vi "CreateDefectFile.vi"(4 "Region":u16, 7 "Pass rate":dbl format="%.2f", 8 "Defect description list":i32[](array[numeric]), 9 "Bad channel array":i32[](array[numeric]), 10 "No of bad strips":i32, 11 "Filename IN":string) -> (0 "DBfileSaved?":bool, 1 "passed":bool)   [LabVIEW 2018]
uses:
  general_VIs/globals/QC_RunInformation.vi
panel:
  in  "cancel":bool
  in  "create file":bool
  out "% good strips:":dbl format="%.2f"
  out "Passed?":bool
  out "ITk Serial No.:":string
  in  "Bad channel list":i32(listbox)
  # "Write Strip Defect DataBase File"
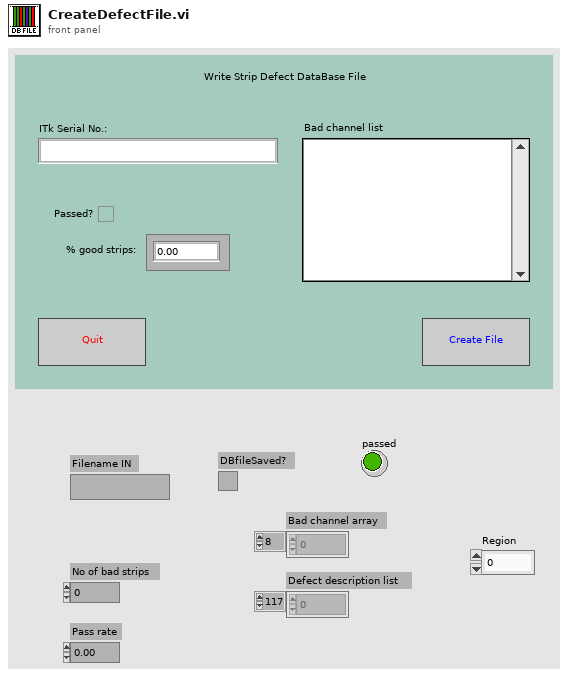
[diagram p1: front panel]
types:
  T1 = cluster{"Institute":string, "Manufacturers":string[], "Devices":string[], "Serialnumbers Lookup DB":string, "Data directory":string, "Backup & screenshot directory":string, "List of known users":string[], "Measurement switch not used":bool, "Measurement Switch":string, "DUT Switch":string, "Rseries IV [MOhm]":string, "Rshunt IV [MOhm]":string, "Rseries CV [MOhm]":string, "DC blocking Cap [µF]":string, "Rseries LCR [MOhm]":string, "Rseries stability [MOhm]":string, "Rshunt stability [MOhm]":string, "Rseries striptest bias [MOhm]":string, "Rseries strip pinhole [MOhm]":string}
  T2 = cluster{"Sensor Serial No.:":string, "Wafer:":string, "Batch:":string, "Manufacturer:":string, "Device Category:":string, "Database Serial No.:":string, "Date Initiated:":string, "Time Initiated:":string, "Test":string, "Probeplan used:":string, "End of Run Status":dbl, "End of Run comment:":string, "User:":string, "Vbias SMU":string, "LCR":string, "Test SMU":string, "Test DMM":string, "Comments":string, "Measurement results":cluster{"IV":string, "CV":string, "Cis":string, "Ris":string, "Stability":string, "PTP":string, "Striptest":string}}
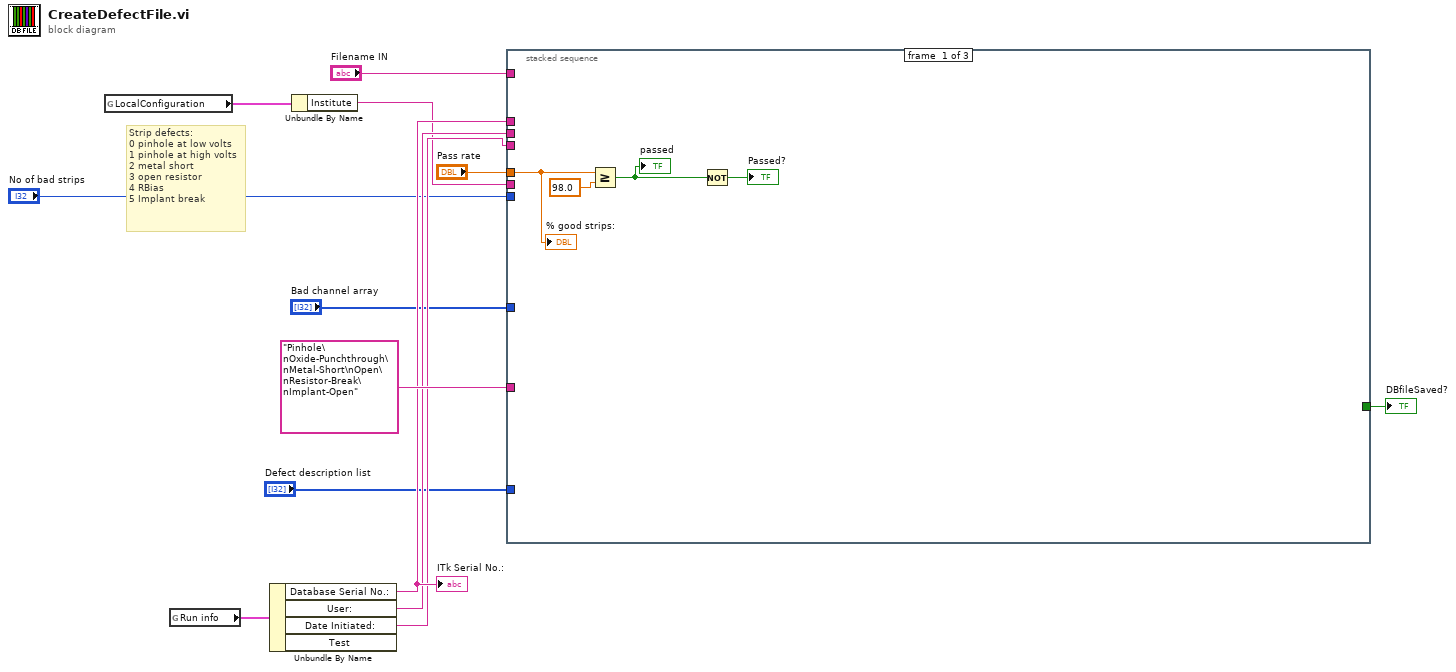
[diagram p0: block diagram]
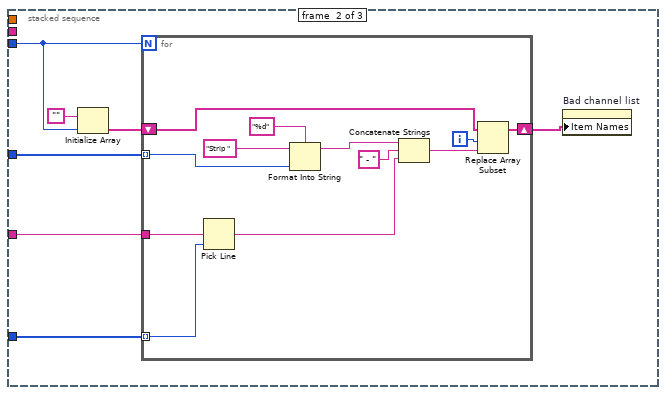
[diagram p2: hidden frame]
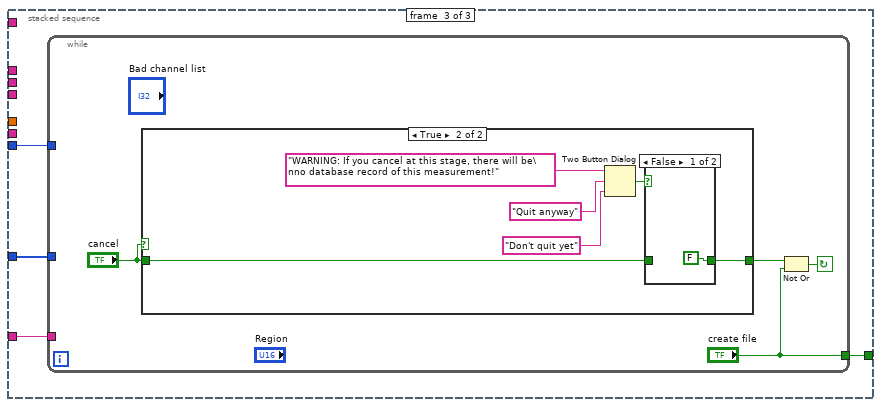
[diagram p3: hidden frame]
diagram:
  # "Strip defects:\n0 pinhole at low volts\n1 pinhole at high volts\n2 metal short\n3 open resistor\n4 RBias\n5 Implant break"
  n1 = global read "QC_RunInformation.vi" "LocalConfiguration"() -> (w2:T1)
  n2 = global read "QC_RunInformation.vi" "Run info"() -> (w12:T2)
  n3 = Unbundle By Name(w12) -> ("Database Serial No.:"=w11:string, "User:"=w10:string, "Date Initiated:"=w9:string)  [unwired: 1 out]
  "ITk Serial No.:" <- w11
  n4 = Unbundle By Name(w2) -> ("Institute"=w1:string)
  n5 = stacked-sequence {
    tunnel: "No of bad strips" -> [_ w18 w39]
    tunnel: "Bad channel array" -> [_ w21 w40]
    tunnel: "Pinhole\nOxide-Punchthrough\nMetal-Short\nOpen\nResistor-Break\nImplant-Open" -> [_ w22 w38]
    tunnel: w11 -> [_ _ _]
    tunnel: w10 -> [_ _ _]
    tunnel: w9 -> [_ _ _]
    tunnel: w1 -> [_ _ _]
    tunnel: [_ _ w37] -> w8
    tunnel: "Filename IN" -> [_ _ _]
    tunnel: "Defect description list" -> [_ w20 _]
    tunnel: "Pass rate" -> [w15 _ _]
    frame #0 {
      n6 = Greater Or Equal?(x=w15, y=98.0) -> (x >= y?=w14:bool)
      "passed" <- w14
      n7 = Not(x=w14) -> (.not. x?=→"Passed?":bool)
      "% good strips:" <- w15
    }
    frame #1 {
      n8 = Initialize Array("", w18) -> (w23:string[])
      n9 = for {
        N: w18 -> [_]
        shift-right: [w31] -> w19
        shift-left: w23 -> [w34]
        tunnel: w21 -> [w25] mode=indexing
        tunnel: w22 -> [w30]
        tunnel: w20 -> [w26] mode=indexing
        i -> [w33]
        n10 = Pick Line(multi-line string=w30, line index=w26) -> (output string=w27:string)  [unwired: 1 in]
        n11 = Format Into String(format string="%d", initial string="Strip ", w25) -> (resulting string=w29:string)  [unwired: 1 in, 1 out]
        n12 = Concatenate Strings(w29, " - ", w27) -> (w32:string)
        n13 = Replace Array Subset(array=w34, new element=w32, index=w33) -> (w31:string[])
      }
      n14 = property on="Bad channel list" class="LstBox (strict)"("Item Names"=w19) -> ()  [unwired: 2 in, 2 out]
    }
    frame #2 {
      n15 = while {
        tunnel: ["create file"] -> w37
        tunnel: w40 -> [_]
        tunnel: w39 -> [_]
        tunnel: w38 -> [_]
        stop <- w44 continue-if-true
        n16 = case shown="True" "cancel" {
          tunnel: [w45 w47] -> w42
          tunnel: "cancel" -> [w45 w46]
          frame False {
          }
          frame True {
            n17 = Two Button Dialog(message="WARNING: If you cancel at this stage, there will be\nno database record of this measurement!", 1:"Don't quit yet" ("F button name (\"Cancel\")"), 2:"Quit anyway" ("T button name (\"OK\")")) -> (T button?=w48:bool)
            n18 = case shown="False" w48 {
              tunnel: [FALSE w53] -> w47
              tunnel: w46 -> [_ w53]
              frame False {
              }
              frame True {
              }
            }
          }
        }
        n19 = Not Or(1:"create file", 2:w42) -> (0:w44:bool)
      }
    }
  }
  "DBfileSaved?" <- w8
